vi "Find events in timeframe.vi"(8 "Data Array":timestamp[](array[timestamp]), 9 "Offset in":i32, 10 "End time":timestamp, 11 "Start time":timestamp) -> (1 "Offset out":i32, 2 "length out":i32, 3 "index out":i32)   [LabVIEW 2011]
panel:
  out "First Element Found":bool
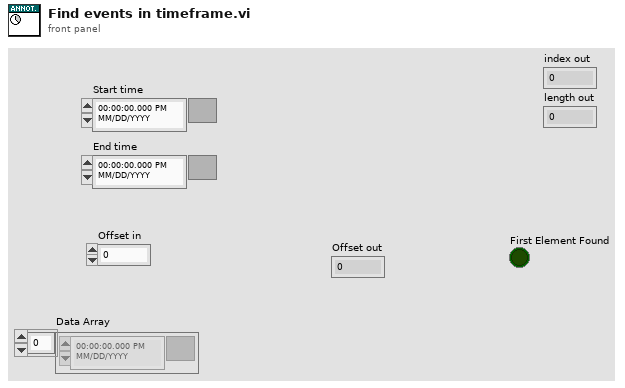
[diagram p1: front panel]
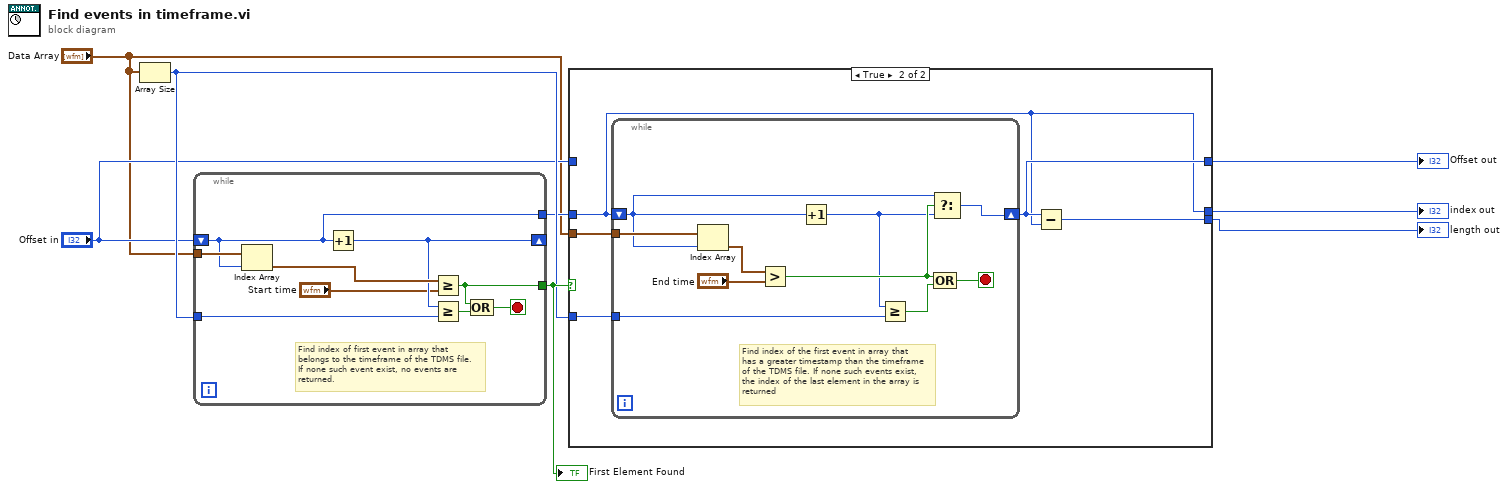
[diagram p0: block diagram]
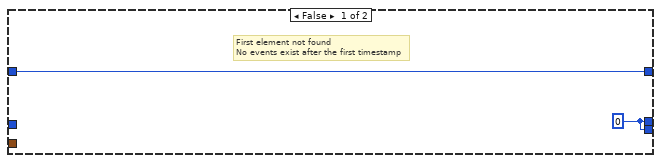
[diagram p2: hidden frame]
diagram:
  n1 = Array Size(array="Data Array") -> (size(s)=w7:i32)
  n2 = while {
    tunnel: "Data Array" -> [w17]
    shift-right: [w14] -> _
    shift-left: "Offset in" -> [w15]
    tunnel: [w15] -> w4
    tunnel: w7 -> [w13]
    tunnel: [w10] -> w8
    stop <- w11 stop-if-true
    # "Find index of first event in array that\nbelongs to the timeframe of the TDMS file.\nIf none such event exist, no events are \nreturned."
    n3 = Index Array(array=w17, index=w15) -> (element=w16:timestamp)
    n4 = Increment(x=w15) -> (x+1=w14:i32)
    n5 = Greater Or Equal?(x=w16, y="Start time") -> (x >= y?=w10:bool)
    n6 = Greater Or Equal?(x=w14, y=w13) -> (x >= y?=w12:bool)
    n7 = Compound Arithmetic op=OR(w10, w12) -> (w11:bool)
  }
  "First Element Found" <- w8
  n8 = case shown="True" w8 {
    tunnel: w4 -> [_ w21]
    tunnel: "Data Array" -> [_ w24]
    tunnel: w7 -> [_ w23]
    tunnel: "Offset in" -> [w19 _]
    tunnel: [w19 w22] -> w5
    tunnel: [w18 w21] -> w3
    tunnel: [w18 w20] -> w2
    frame False {
      w18 = 0 ("Starting index")
      # "First element not found\nNo events exist after the first timestamp"
    }
    frame True {
      n9 = while {
        shift-right: [w26] -> w22
        shift-left: w21 -> [w28]
        tunnel: w24 -> [w33]
        tunnel: w23 -> [w31]
        stop <- w30 stop-if-true
        # "Find index of the first event in array that\nhas a greater timestamp than the timeframe\nof the TDMS file. If none such events exist, \nthe index of the last element in the array is \nreturned"
        n10 = Index Array(array=w33, index=w28) -> (element=w34:timestamp)
        n11 = Greater?(x=w34, y="End time") -> (0:w29:bool)
        n12 = Increment(x=w28) -> (x+1=w27:i32)
        n13 = Greater Or Equal?(x=w27, y=w31) -> (x >= y?=w32:bool)
        n14 = Select(t=w28, s=w29, f=w27) -> (s? t:f=w26:i32)
        n15 = Compound Arithmetic op=OR(w29, w32) -> (w30:bool)
      }
      n16 = Subtract(x=w22, y=w21) -> (x-y=w20:i32)
    }
  }
  "Offset out" <- w5
  "index out" <- w3
  "length out" <- w2
